vi "STD电导率_获取温度和测量值.vi"(8 "error in (no error)":errorcluster caption="错误输入（无错误）", 11 "MB session in":refnum<class "MB_Master.lvclass">) -> (0 "error out":errorcluster caption="错误输出", 2 "STDspcond":cluster{"温度测量值":sgl, "测量值":sgl, "信号值":sgl}, 3 "MB session out":refnum<class "MB_Master.lvclass">)   [LabVIEW 2016, in "斯坦道多参数.lvlib"]
uses:
  <vilib>/Plasmionique/MB Master/MB_Master/MB_Master.lvclass
  <vilib>/Plasmionique/MB Master/MB Master.lvlib
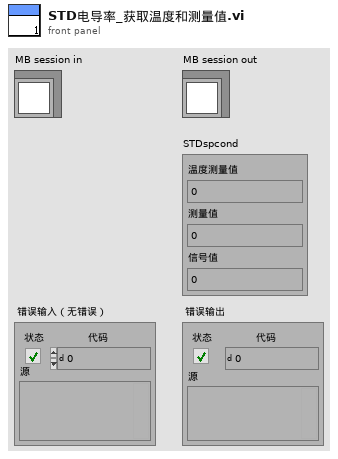
[diagram p1: front panel]
types:
  T1 = cluster{"pH":u32, "DO":u32, "Cond":u32, "Turb":u32, "叶绿素a":u32, "藻密度":u32, "ORP":u32, "COD":u32, "氯化物":u32, "氨氮":u32, "水中油":u32}
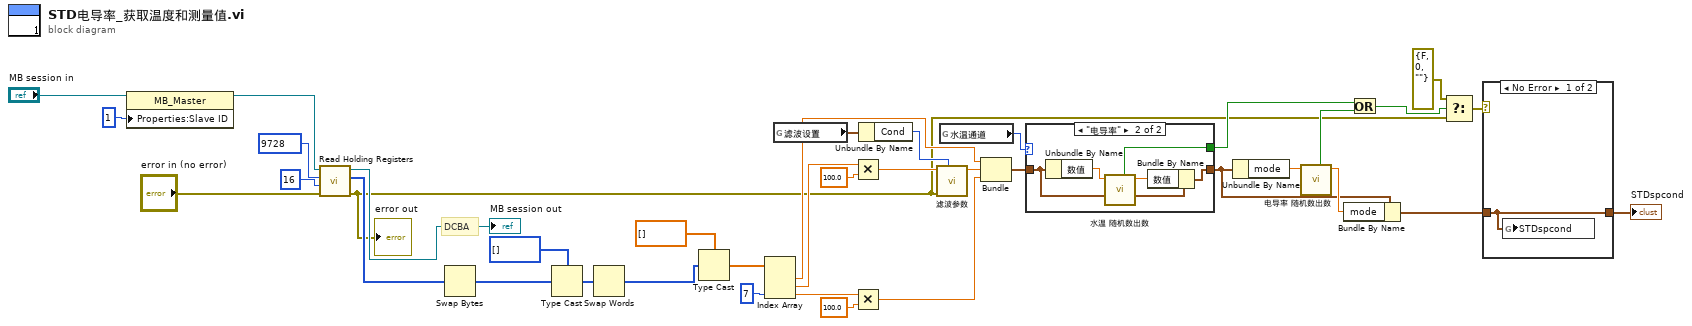
[diagram p0: block diagram]
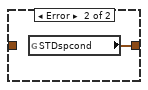
[diagram p3: hidden frame]
diagram:
  # "DCBA"
  n1 = property class="MB_Master"(reference="MB session in", "Properties:Slave ID"=u16 1 ("y")) -> (reference out=w30:refnum<class "MB_Master.lvclass">)  [unwired: 1 in, 1 out]
  n2 = call <vilib>:"Read Holding Registers.vi"("error in (no error)"="error in (no error)", "quantity"=u16 16, "starting address"=u16 9728, "MB session in"=w30) -> ("error out"=w3:errorcluster, "Registers"=w28:u16[], "MB session out"=→"MB session out":refnum<class "MB_Master.lvclass">)  [unwired: 5 in]
  "error out" <- w3
  n3 = Swap Bytes(anything=w28) -> (byte swapped=w17:u16[])
  n4 = Type Cast(type=u32[] [] ("数组 2"), x=w17) -> (*(type *) &x=w34:u32[])
  n5 = Swap Words(1:w34) -> (0:w36:u32[])
  n6 = Type Cast(type=sgl[] [] ("数组 2"), x=w36) -> (*(type *) &x=w32:sgl[])
  n7 = Index Array(array=w32, index #3=7 ("索引")) -> (element #1=w27:sgl, element #2=w26:sgl, element #3=w15:sgl)  [unwired: 2 in]
  n8 = global read "断电保存变量.vi" "滤波设置"() -> (w20:T1)
  n9 = Multiply(x=w26, y=sgl 100.0) -> (x*y=w22:sgl)
  n10 = Multiply(x=w15, y=sgl 100.0) -> (x*y=w14:sgl)
  n11 = Unbundle By Name(w20) -> ("Cond"=w19:u32)
  n12 = call "滤波参数.vi"("滤波次数"=w19, "error in (no error)"=w3, "x"=w22) -> ("mode"=w21:dbl)  [unwired: 7 in, 1 out]
  n13 = global read "断电保存变量.vi" "水温通道"() -> (w11:enum16{"pH", "DO", "浊度", "电导率", "叶绿素a", "藻密度"})
  n14 = Bundle("数值"=w27, "mode"=w21, w14) -> (w10:cluster{"数值":sgl, "mode":dbl, sgl})  [unwired: 1 in]
  n15 = case shown="\"电导率\"" w11 {
    tunnel: w10 -> [w39 w43]
    tunnel: [w39 w41] -> w8
    tunnel: [_ w40] -> w6
    frame Default {
    }
    frame "电导率" {
      n16 = Unbundle By Name(w43) -> ("数值"=w44:sgl)
      n17 = call "水温 随机数出数.vi"("原始值"=w44) -> ("取值输出"=w42:dbl, "x .and. y?"=w40:bool)  [unwired: 6 in, 1 out]
      n18 = Bundle By Name(cluster=w43, "数值"=w42) -> (w41:cluster{"数值":sgl, "mode":dbl, sgl})
    }
  }
  n19 = Unbundle By Name(w8) -> ("mode"=w13:dbl)
  n20 = call "电导率 随机数出数.vi"("原始值"=w13) -> ("取值输出"=w12:dbl, "x .and. y?"=w5:bool)  [unwired: 6 in, 1 out]
  n21 = Bundle By Name(cluster=w8, "mode"=w12) -> (w7:cluster{"数值":sgl, "mode":dbl, sgl})
  n22 = Or(x=w6, y=w5) -> (x .or. y?=w4:bool)
  n23 = Select(t=errorcluster {"status"=FALSE, "code"=0, "source"=""}, s=w4, f=w3) -> (s? t:f=w2:errorcluster)
  n24 = case shown="No Error" w2 {
    tunnel: w7 -> [w45 _]
    tunnel: [w45 w46] -> w9
    frame No Error {
      n25 = global write "禹山过程全局变量.vi" "STDspcond"(w45) -> ()
    }
    frame Error {
      n26 = global read "禹山过程全局变量.vi" "STDspcond"() -> (w46:cluster{"温度测量值":sgl, "测量值":sgl, "信号值":sgl})
    }
  }
  "STDspcond" <- w9
